vi "dfd_Evaluate N(z) Over D(z).vi"(1 "w":dbl format="%.2f", 2 "D(z)":cluster{"Di(z)":dbl[]}[](array[cluster]) {"Di(z)" format="%.4f"}, 3 "N(z)":cluster{"Ni(z)":dbl[]}[](array[cluster]) {"Ni(z)" format="%.4f"}) -> (0 "H(exp(jw))":cdb format="%.4f")   [LabVIEW 2017, in "NI_DigFilter_Design.lvlib"]
uses:
  <vilib>/addons/Digital Filter Design/NI_DigFilter_Design.lvlib
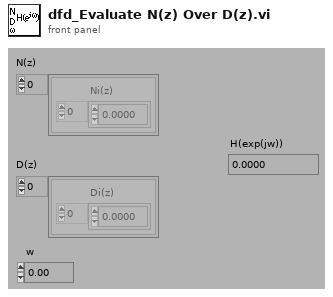
[diagram p1: front panel]
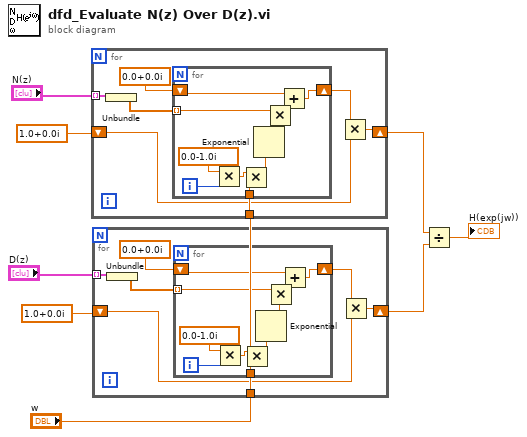
[diagram p0: block diagram]
diagram:
  n1 = for {
    tunnel: "N(z)" -> [w15] mode=indexing
    shift-right: [w12] -> w3
    shift-left: cdb 1.0+0.0i -> [w11]
    tunnel: "w" -> [w13]
    n2 = Unbundle(w15) -> ("Ni(z)"=w14:dbl[])
    n3 = for {
      shift-right: [w20] -> w9
      shift-left: cdb 0.0+0.0i -> [w18]
      tunnel: w14 -> [w17] mode=indexing
      tunnel: w13 -> [w16]
      i -> [w25]
      n4 = Multiply(x=cdb 0.0-1.0i, y=w25) -> (x*y=w23:cdb)
      n5 = Multiply(x=w23, y=w16) -> (x*y=w22:cdb)
      n6 = Exponential(1:w22) -> (0:w21:cdb)
      n7 = Multiply(x=w17, y=w21) -> (x*y=w19:cdb)
      n8 = Add(x=w18, y=w19) -> (x+y=w20:cdb)
    }
    n9 = Multiply(x=w9, y=w11) -> (x*y=w12:cdb)
  }
  n10 = for {
    tunnel: "D(z)" -> [w32] mode=indexing
    shift-right: [w28] -> w2
    shift-left: cdb 1.0+0.0i -> [w27]
    tunnel: "w" -> [w30]
    n11 = Unbundle(w32) -> ("Di(z)"=w31:dbl[])
    n12 = for {
      shift-right: [w37] -> w29
      shift-left: cdb 0.0+0.0i -> [w35]
      tunnel: w31 -> [w34] mode=indexing
      tunnel: w30 -> [w33]
      i -> [w42]
      n13 = Multiply(x=cdb 0.0-1.0i, y=w42) -> (x*y=w40:cdb)
      n14 = Multiply(x=w40, y=w33) -> (x*y=w39:cdb)
      n15 = Exponential(1:w39) -> (0:w38:cdb)
      n16 = Multiply(x=w34, y=w38) -> (x*y=w36:cdb)
      n17 = Add(x=w35, y=w36) -> (x+y=w37:cdb)
    }
    n18 = Multiply(x=w29, y=w27) -> (x*y=w28:cdb)
  }
  n19 = Divide(x=w3, y=w2) -> (x/y=→"H(exp(jw))":cdb)
